vi "Edit calibration.vi"(2 "Ports":T1, 3 "Data Display":T3 {"average data rate (Hz)" format="%.2f"; "Min Range" format="%.3f"; "Max Range" format="%.3f"; "Mean (Volts)" format="%.5f"; "Mean (scaled)" format="%.2f"}, 4 "Index":u32) -> ()   [LabVIEW 2012]
uses:
  conversion.ctl
  DAQ configuration/scale type.ctl
  correspondence table.ctl
  pH/pH scale.ctl
  Dissolved Oxygen/DO scale.ctl
  calibrator graph.ctl
  DAQ configuration/Sensor array.ctl
  DAQ configuration/channel identifier.ctl
  global scale array.vi
  <vilib>/Analysis/1siggen.llb/Ramp Pattern by Samples.vi
  <vilib>/Analysis/NI_AALBase.lvlib
panel:
  out "Calibration Graph":cluster{"Ramp Pattern":dbl[], sgl[]}(graph)
  out "Calibration in":T4 {"D.O."."K" format="%.6f"; "D.O."."Temperature" format="%.2f"; "pH scale"."Buffers"."V/T" format="%.5f"; "pH scale"."Buffers"."Buffer" format="%.2f"; "pH scale"."Temperature" format="%.2f"; "offset (physical units)" format="%.5f"; "correspondence table"."volts" format="%.4f"; "correspondence table"."physical units" format="%.4f"; "second channel" min=-1; "offset (volts)" format="%.5f"; "conversion matrix" format="%.4e"}
  in  "Cancel Button":bool
  in  "OK Button":bool
  in  "Calibration":T4 {"D.O."."K" format="%.6f"; "D.O."."Temperature" format="%.2f"; "pH scale"."Buffers"."V/T" format="%.5f"; "pH scale"."Buffers"."Buffer" format="%.2f"; "pH scale"."Temperature" format="%.2f"; "offset (physical units)" format="%.5f"; "correspondence table"."volts" format="%.4f"; "correspondence table"."physical units" format="%.4f"; "second channel" min=-1; "offset (volts)" format="%.5f"; "conversion matrix" format="%.4e"}
  # "V"
  # "V"
  # "C"
  # "kPa"
  # "C"
  # "C"
  # "kPa"
  # "C"
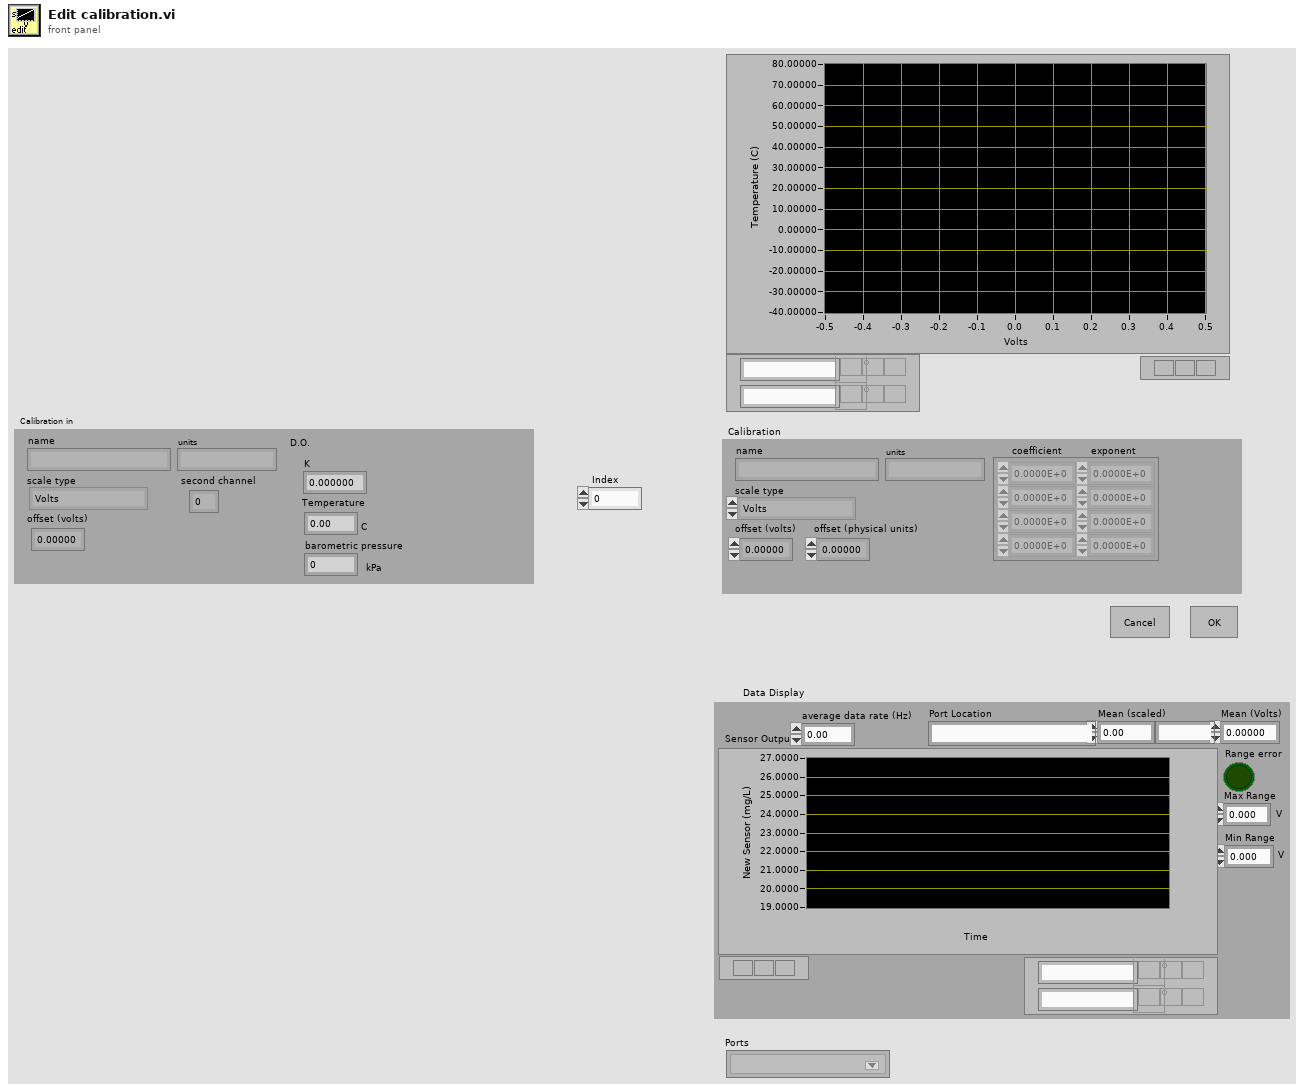
[diagram p1: front panel]
types:
  T1 = typedef "Sensor array.ctl" = T2[]
  T2 = typedef "channel identifier.ctl" = u16
  T3 = typedef "calibrator graph.ctl" = cluster{"Range error":bool, "Mean (scaled)":dbl, "Mean (Volts)":dbl, "Max Range":dbl, "Min Range":dbl, "units":string, "Sensor Output":cluster{dbl[], dbl[]}[], "Port Location":string, "average data rate (Hz)":dbl}
  T4 = typedef "conversion.ctl" = cluster{"conversion matrix":sgl[][], "units":string, "name":string, "scale type":T5, "offset (volts)":dbl, "second channel":i8, "correspondence table":T6, "offset (physical units)":dbl, "pH scale":T7, "D.O.":T8}
  T5 = typedef "scale type.ctl" = enum16{"Volts", "Polynomial", "Correspondence Table", "pH", "Dissolved Oxygen", "Quadratic"}
  T6 = typedef "correspondence table.ctl" = cluster{"physical units":dbl, "volts":dbl}[]
  T7 = typedef "pH scale.ctl" = cluster{"Buffers":cluster{"Buffer":dbl, "Calibrated":bool, "V/T":dbl}[], "Temperature":dbl}
  T8 = typedef "DO scale.ctl" = cluster{"Temperature":dbl, "K":dbl, "barometric pressure":dbl}
  T9 = typedef "calib array.ctl" = T4[]
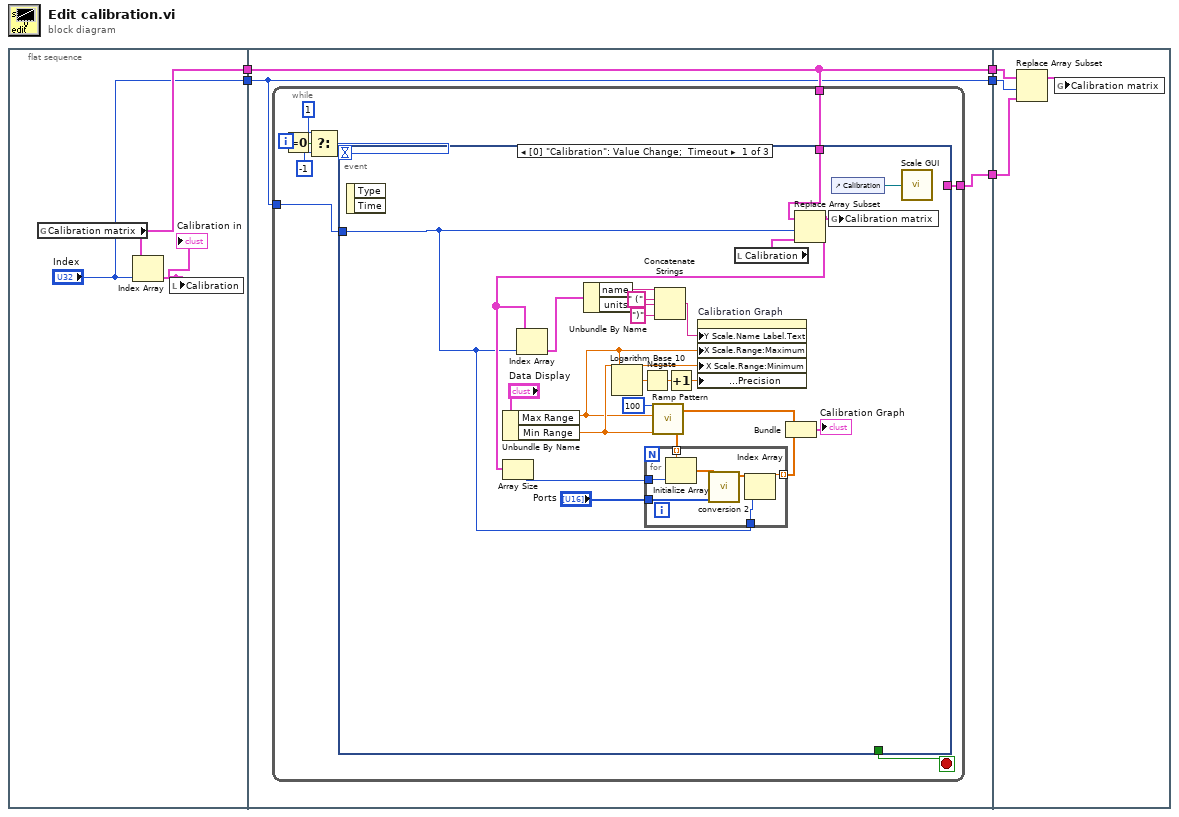
[diagram p0: block diagram]
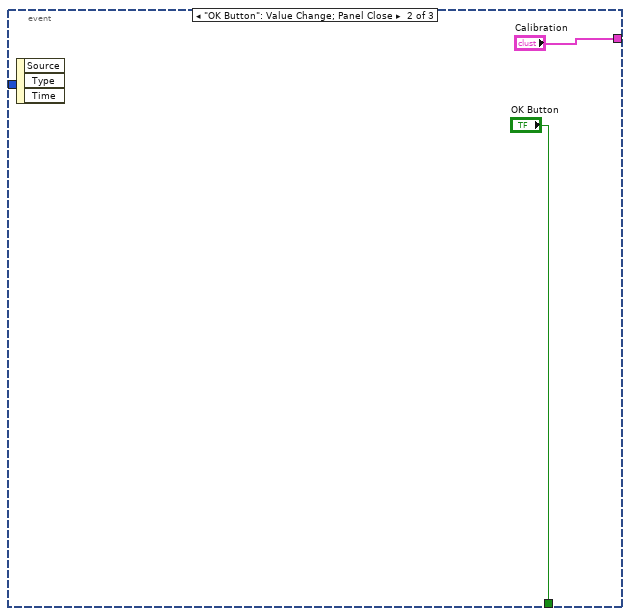
[diagram p2: hidden frame]
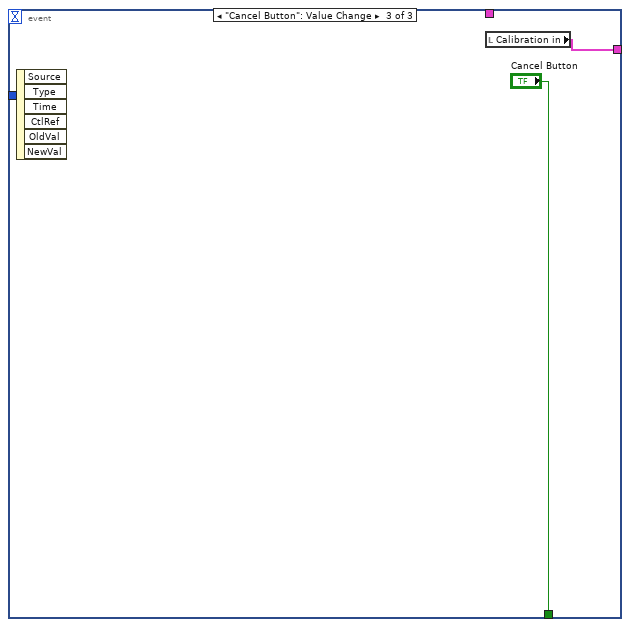
[diagram p3: hidden frame]
diagram:
  n1 = flat-sequence {
    tunnel: [w7] -> w4
    tunnel: ["Index"] -> w2
    tunnel: [w10] -> w5
    tunnel: w4 -> [w10]
    tunnel: [w9] -> w3
    tunnel: w2 -> [w9]
    tunnel: [w11] -> w1
    tunnel: w5 -> [w57]
    tunnel: w3 -> [w56]
    tunnel: w1 -> [w55]
    frame #0 {
      n2 = global read "global scale array.vi" "Calibration matrix"() -> (w7:T9)
      n3 = Index Array(array=w7, index="Index") -> (element=w8:T4)
      "Calibration in" <- w8
      n4 = local write "Calibration"(w8) -> ()
    }
    frame #1 {
      n5 = while {
        tunnel: [w20] -> w11
        tunnel: w10 -> [w13]
        tunnel: w9 -> [w12]
        i -> [w15]
        stop <- w19 stop-if-true
        n6 = Equal To 0?(x=w15) -> (x = 0?=w14:bool)
        n7 = Select(t=1, s=w14, f=-1) -> (s? t:f=w16:i32)
        n8 = event shown="[0] \"Calibration\": Value Change;  Timeout" {
          selector: _ -> [_ _ _]
          dyn-events: _ -> [_ _ _]
          timeout: w16 -> [_ _ _]
          tunnel: [_ "Calibration" w53] -> w20
          tunnel: [_ "OK Button" "Cancel Button"] -> w19
          tunnel: w13 -> [w41 _ _]
          tunnel: w12 -> [w22 _ _]
          event Value Change; Timeout {
            n9 = event-data() -> ()  [unwired: 1 in, 2 out]
            n10 = Unbundle By Name("Data Display") -> ("Max Range"=w28:dbl, "Min Range"=w30:dbl)
            n11 = Logarithm Base 10(1:w28) -> (0:w29:dbl)
            n12 = Negate(x=w29) -> (-x=w27:dbl)
            n13 = call-poly <vilib>:"Ramp Pattern.vi"("start"=w30, "end"=w28, "samples"=100) -> ("Ramp Pattern"=w38:dbl[])  [unwired: 7 in, 1 out]
            n14 = Increment(x=w27) -> (x+1=w26:dbl)
            n15 = local read "Calibration"() -> (w42:T4)
            n16 = Replace Array Subset(array=w41, new element=w42, index=w22) -> (w23:T9)
            n17 = Array Size(array=w23) -> (size(s)=w24:i32)
            n18 = Index Array(array=w23, index=w22) -> (element=w36:T4)
            n19 = Unbundle By Name(w36) -> ("name"=w35:string, "units"=w33:string)
            n20 = for {
              tunnel: w38 -> [w48] mode=indexing
              tunnel: [w49] -> w25 mode=indexing
              tunnel: w24 -> [w47]
              tunnel: w22 -> [w45]
              tunnel: "Ports" -> [w44]
              n21 = Initialize Array(w48, w47) -> (w46:dbl[])
              n22 = call "conversion 2.vi"("Channel Indices"=w44, "voltage data"=w46) -> ("calibrated data"=w50:sgl[])  [unwired: 8 in, 1 out]
              n23 = Index Array(array=w50, index=w45) -> (element=w49:sgl)
            }
            n24 = Concatenate Strings(w35, " (" ("Substring"), w33, ")" ("Substring")) -> (w31:string)
            n25 = property on="Calibration Graph" class="XYGraph (strict)"("Y Scale.Name Label.Text"=w31, "X Scale.Range:Maximum"=w28, "X Scale.Range:Minimum"=w30, "X Scale.Format & Precision:Precision"=w26) -> ()  [unwired: 2 in, 2 out]
            n26 = Bundle("Ramp Pattern"=w38, w25) -> (→"Calibration Graph":cluster{"Ramp Pattern":dbl[], sgl[]})  [unwired: 1 in]
            n27 = global write "global scale array.vi" "Calibration matrix"(w23) -> ()
            n28 = control-ref of="Calibration"() -> (w43:refnum<vi>)
            n29 = call "Scale GUI.vi"("Clust Refnum"=w43) -> ()
          }
          event "OK Button": Value Change; Panel Close {
            n30 = event-data() -> ()  [unwired: 1 in, 3 out]
          }
          event "Cancel Button": Value Change {
            n31 = event-data() -> ()  [unwired: 1 in, 6 out]
            n32 = local read "Calibration in"() -> (w53:T4)
          }
        }
      }
    }
    frame #2 {
      n33 = Replace Array Subset(array=w57, new element=w55, index=w56) -> (w58:T9)
      n34 = global write "global scale array.vi" "Calibration matrix"(w58) -> ()
    }
  }
